vi "Cache-CSMKVMapDVR.vi"() -> (3 "KVMapDVR":refnum<data-value>)   [LabVIEW 2017, in "Communicable State Machine.lvlib"]
uses:
  Communicable State Machine.lvlib
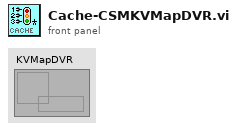
[diagram p1: front panel]
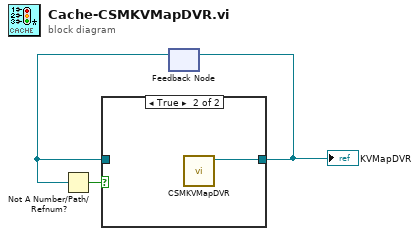
[diagram p0: block diagram]
diagram:
  n1 = feedback #1() -> (w1:refnum<data-value>)  [unwired: 1 in]
  n2 = Not A Number/Path/Refnum?(number/path/refnum=w1) -> (NaN/Path/Refnum?=w2:bool)
  n3 = case shown="True" w2 {
    tunnel: w1 -> [w4 _]
    tunnel: [w4 w5] -> w3
    frame False {
    }
    frame True {
      n4 = call "CSMKVMapDVR.vi"() -> ("KVMapDVR"=w5:refnum<data-value>)  [unwired: 11 in]
    }
  }
  "KVMapDVR" <- w3
  n5 = feedback-in #1(w3) -> ()
